vi "GE 5565PIORC.PIO.Read In-Place (U8).vi"(8 "error in (no error)":errorcluster, 9 "data in":u8, 10 "offset":u32, 11 "GE 5565PIORC in":refnum<class "GE 5565PIORC.lvclass">) -> (0 "error out":errorcluster, 1 "data out":u8, 3 "GE 5565PIORC out":refnum<class "GE 5565PIORC.lvclass">)   [LabVIEW 2020, in "GE 5565PIORC.lvclass"]
doc: "Reads from the specified <B>offset</B> and places the contents into <B>data</B>."
uses:
  GE 5565PIORC.lvclass
  <vilib>/Instr/_visa.llb/VISA Register Access Address Space.ctl
  GE 5565PIORC.lvclass/GE 5565PIORC.ctl
  GE 5565PIORC.VISA.Move In-Place.String (U8).vi
  GE 5565PIORC.VISA.Return Handler.vi
  <vilib>/Utility/error.llb/Error Cluster From Error Code.vi
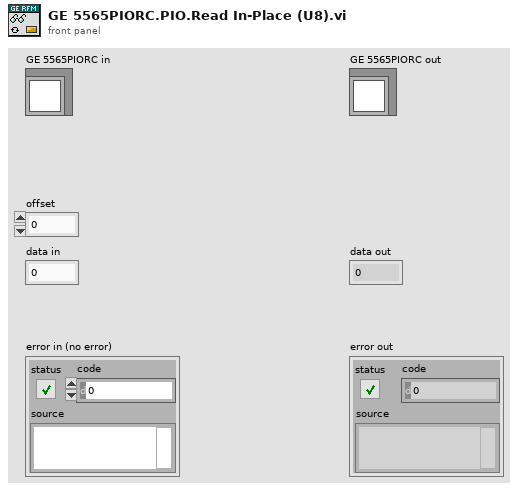
[diagram p1: front panel]
types:
  T1 = typedef "VISA Register Access Address Space.ctl" = u16
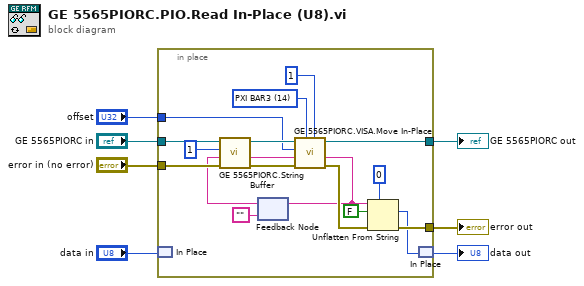
[diagram p0: block diagram]
diagram:
  n1 = in-place {
    in-place-border: "error in (no error)" -> [w18]
    in-place-border: [w25] -> w6
    in-place-border: "GE 5565PIORC in" -> [w19]
    in-place-border: "offset" -> [w12]
    in-place-border: [w22] -> w3
    w23 = T1 14 items=["VXI/VME A16"=1, "VXI/VME A24"=2, "VXI/VME A32"=3, "VXI/VME A64"=4, "PXI Memory Allocations"=9, "PXI Configuration"=10, "PXI BAR0"=11, "PXI BAR1"=12, "PXI BAR2"=13, "PXI BAR3"=14, "PXI BAR4"=15, "PXI BAR5"=16] ("address space")
    n2 = in-place-match #1("data in") -> ()  [unwired: 1 out]
    n3 = feedback #2("" ("data out")) -> (w14:string)
    n4 = call "GE 5565PIORC.String Buffer.vi"("error in (no error)"=w18, "string buffer in"=w14, "minimum size"=1, "GE 5565PIORC in"=w19) -> ("error out"=w17:errorcluster, "string buffer out"=w16:string, "GE 5565PIORC out"=w20:refnum<class "GE 5565PIORC.lvclass">)  [unwired: 5 in]
    n5 = call-poly "GE 5565PIORC.VISA.Move In-Place.vi"("count (-1: all)"=1, "address space"=w23, "error in (no error)"=w17, "data in"=w16, "offset"=w12, "GE 5565PIORC in"=w20) -> ("error out"=w21:errorcluster, "data out"=w15:string, "GE 5565PIORC out"=w22:refnum<class "GE 5565PIORC.lvclass">)  [unwired: 3 in]
    n6 = feedback-in #2(w15) -> ()
    n7 = Unflatten From String(type=u8 0, binary string=w15, data includes array or string size? (T)=FALSE, error in (no error)=w21) -> (value=w11:u8, error out=w25:errorcluster)  [unwired: 1 in, 1 out]
    n8 = in-place-match #1(w11) -> (→"data out":u8)
  }
  "GE 5565PIORC out" <- w3
  "error out" <- w6
